vi "Add Entry.vi"(8 "error in (no error)":errorcluster, 9 "Value":variant, 10 "Key":string caption="Name", 11 "Registry in":refnum<class "Registry.lvclass">) -> (0 "error out":errorcluster, 2 "Replaced?":bool, 3 "Registry out":refnum<class "Registry.lvclass">)   [LabVIEW 2020, in "BCI-1553 API.lvlib" / "Registry.lvlib" / "Registry.lvclass"]
doc: "Add a Key/Value pair to the Registry."
uses:
  Registry.lvclass
  Registry.lvclass/Registry.ctl
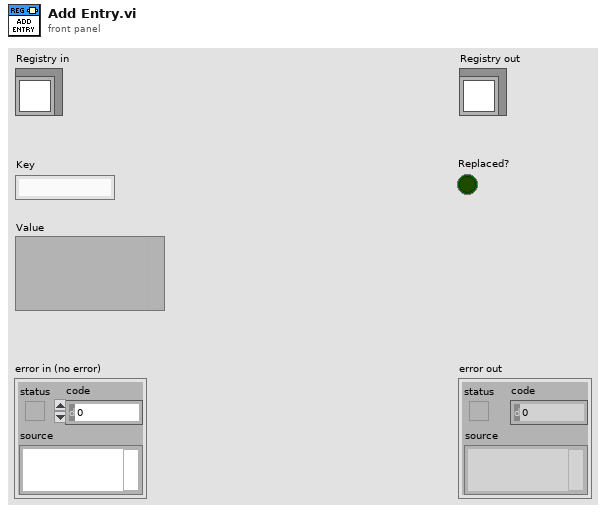
[diagram p1: front panel]
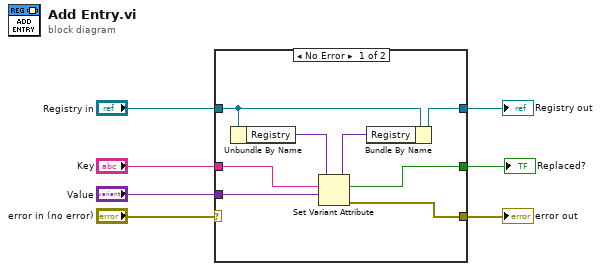
[diagram p0: block diagram]
diagram:
  n1 = case shown="No Error" "error in (no error)" {
    selector: "error in (no error)" -> [_ w17]
    tunnel: [w12 w17] -> w6
    tunnel: [w8 w16] -> w4
    tunnel: "Registry in" -> [w9 w16]
    tunnel: "Key" -> [w15 _]
    tunnel: "Value" -> [w14 _]
    tunnel: [w13 _] -> w2
    frame No Error {
      n2 = Unbundle By Name(w9) -> ("Registry"=w11:variant)
      n3 = Set Variant Attribute(Variant=w11, name=w15, value=w14) -> (Variant out=w10:variant, replaced=w13:bool, error out=w12:errorcluster)  [unwired: 1 in]
      n4 = Bundle By Name(cluster=w9, "Registry"=w10) -> (w8:refnum<class "Registry.lvclass">)
    }
    frame Error {
    }
  }
  "error out" <- w6
  "Registry out" <- w4
  "Replaced?" <- w2
